vi "real64_log10_array.vi"(11 "values":dbl[](array[numeric])) -> (3 "log_values":dbl[](array[numeric]))   [LabVIEW 2020]
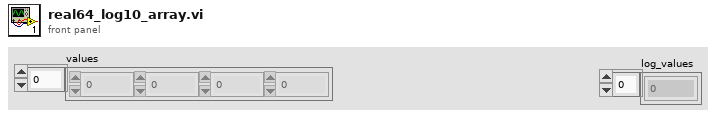
[diagram p1: front panel]
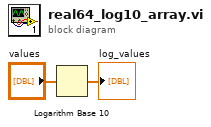
[diagram p0: block diagram]
diagram:
  n1 = Logarithm Base 10(1:"values") -> (0:→"log_values":dbl[])
